vi "String to string array.vi"(10 "delimiter (\\)":string="\\", 11 "String":string) -> (3 "Array":string[](array[string]))   [LabVIEW 2020, in "Blue Tree Map OpenSource.lvlib"]
uses:
  Blue Tree Map OpenSource.lvlib
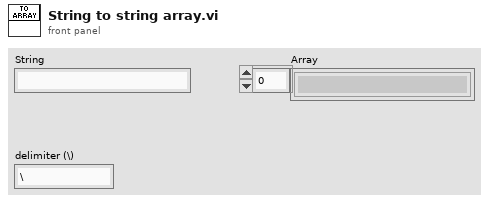
[diagram p1: front panel]
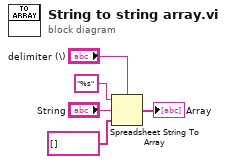
[diagram p0: block diagram]
diagram:
  n1 = Spreadsheet String To Array(delimiter (Tab)="delimiter (\\)", format string="%s", spreadsheet string="String", array type (2D Dbl)=string[] []) -> (array=→"Array":string[])
